vi "Release ChnlHits Semaphore.vi"(3 "Refnum out":T1, 8 "error in (no error)":errorcluster) -> (0 "error out":errorcluster)   [LabVIEW 2016]
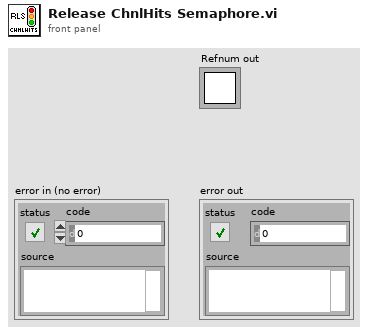
[diagram p1: front panel]
types:
  T1 = typedef "Semaphore RefNum" = refnum<k1>
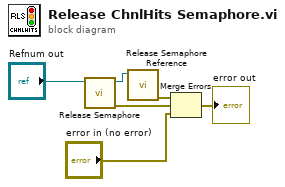
[diagram p0: block diagram]
diagram:
  n1 = call <vilib>:"Release Semaphore.vi"("semaphore"="Refnum out") -> ("error out"=w3:errorcluster, "semaphore out"=w6:T1)  [unwired: 5 in]
  n2 = call <vilib>:"Release Semaphore Reference.vi"("semaphore"=w6) -> ("error out"=w4:errorcluster)  [unwired: 9 in, 1 out]
  n3 = Merge Errors(w4, w3, "error in (no error)") -> (→"error out":errorcluster)
